vi "setClaseProducto.vi"(6 "error in":errorcluster, 8 "Cluster of class private data":T1, 9 "claseProducto in":refnum<class "claseProducto.lvclass">) -> (0 "error out":errorcluster, 3 "claseProducto out":refnum<class "claseProducto.lvclass">)   [LabVIEW 2014, in "claseProducto.lvclass"]
uses:
  claseProducto.lvclass
  claseProducto.lvclass/claseProducto.ctl
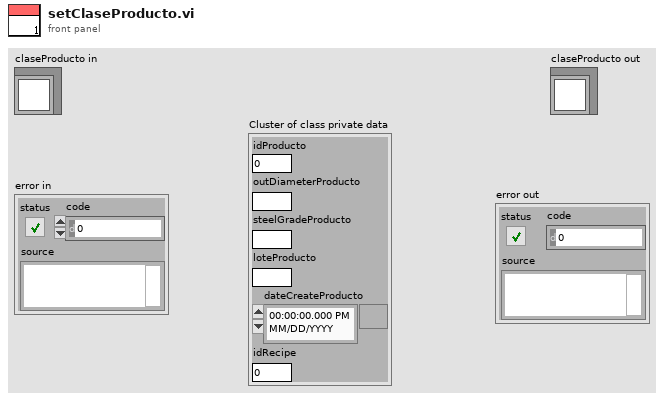
[diagram p1: front panel]
types:
  T1 = cluster{"idProducto":dbl, "outDiameterProducto":string, "steelGradeProducto":string, "loteProducto":string, "dateCreateProducto":timestamp, "idRecipe":dbl}
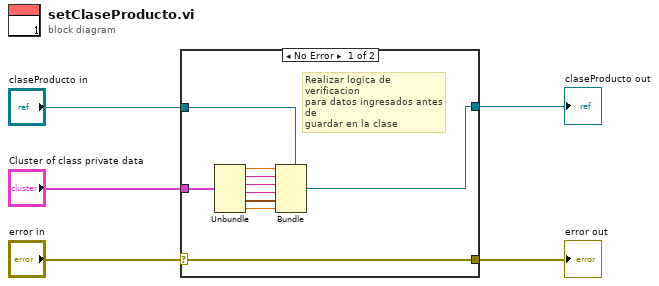
[diagram p0: block diagram]
diagram:
  n1 = case shown="No Error" "error in" {
    selector: "error in" -> [w6 w17]
    tunnel: [w6 w17] -> w4
    tunnel: "claseProducto in" -> [w15 w16]
    tunnel: [w7 w16] -> w2
    tunnel: "Cluster of class private data" -> [w14 _]
    frame No Error {
      # "Realizar logica de verificacion\npara datos ingresados antes de\nguardar en la clase"
      n2 = Unbundle(w14) -> ("idProducto"=w13:dbl, "outDiameterProducto"=w12:string, "steelGradeProducto"=w11:string, "loteProducto"=w10:string, "dateCreateProducto"=w9:timestamp, "idRecipe"=w8:dbl)
      n3 = Bundle(cluster=w15, w13, w12, w11, w10, w9, w8) -> (w7:refnum<class "claseProducto.lvclass">)
    }
    frame Error {
    }
  }
  "claseProducto out" <- w2
  "error out" <- w4
